vi "Timer Action Engine Auto Reset.vi"(9 "Current State":bool, 10 "Time Duration (s)":dbl, 11 "Action":T1) -> (0 "Quit Timer":bool, 1 "Clock Output":bool, 2 "Pulse Out":bool, 3 "Time Elapsed":dbl)   [LabVIEW 2021]
uses:
  Controls/Timer Actions.ctl
panel:
  # "Momentary Pulse O/P"
  # "Square Wave Pulse O/P"
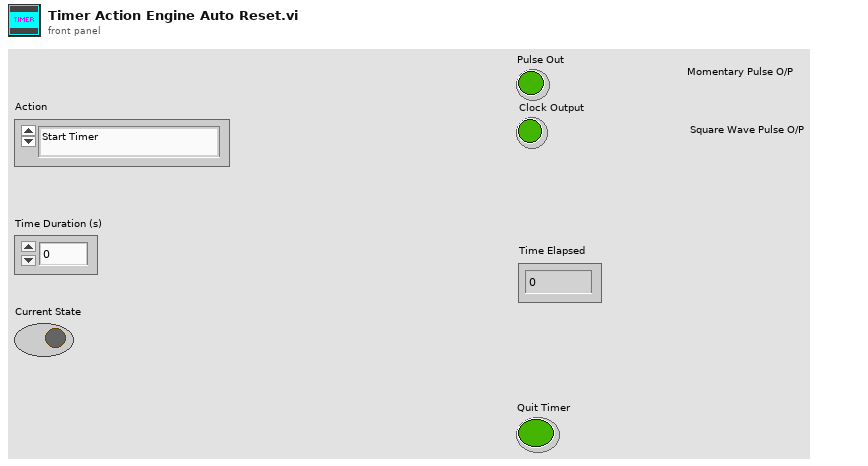
[diagram p1: front panel]
types:
  T1 = typedef "Timer Actions.ctl" = enum16{"Start Timer", "Restart Timer", "Check Timer", "Pause Timer", "Reset Timer", "Exit Timer"}
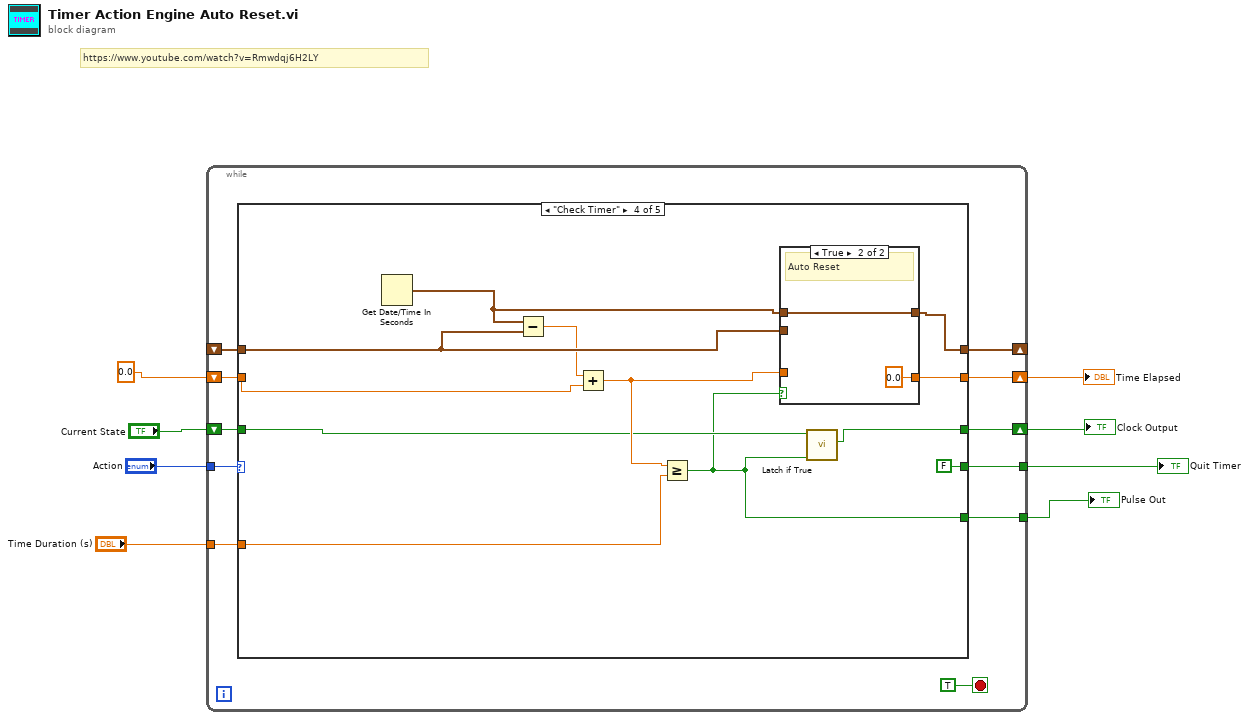
[diagram p0: block diagram]
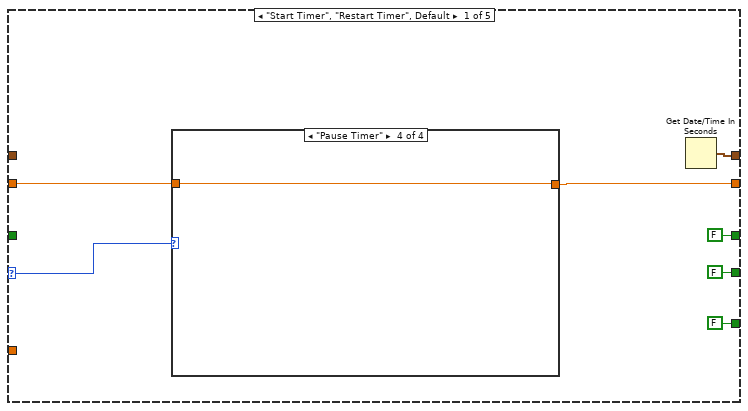
[diagram p2: hidden frame]
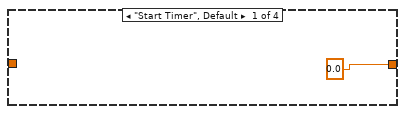
[diagram p3: hidden frame]
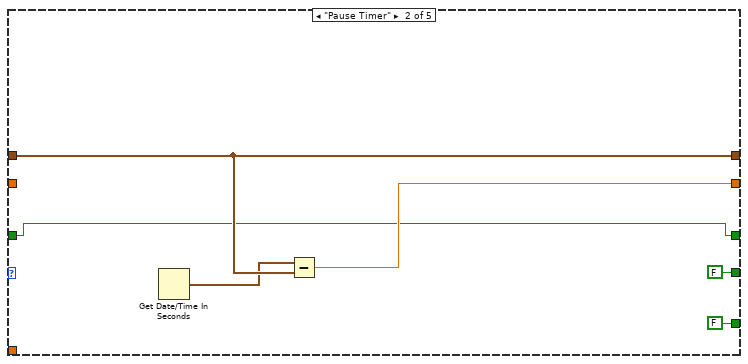
[diagram p6: hidden frame]
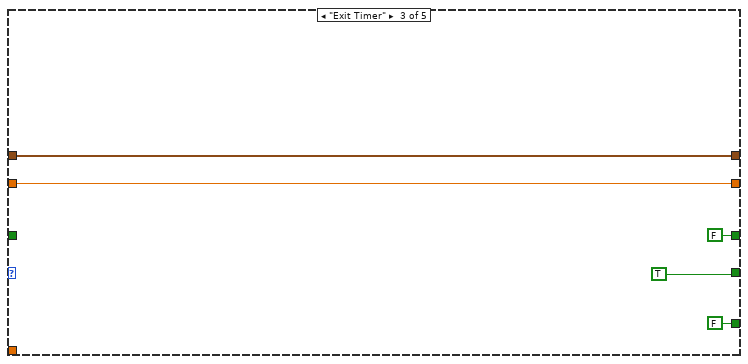
[diagram p7: hidden frame]
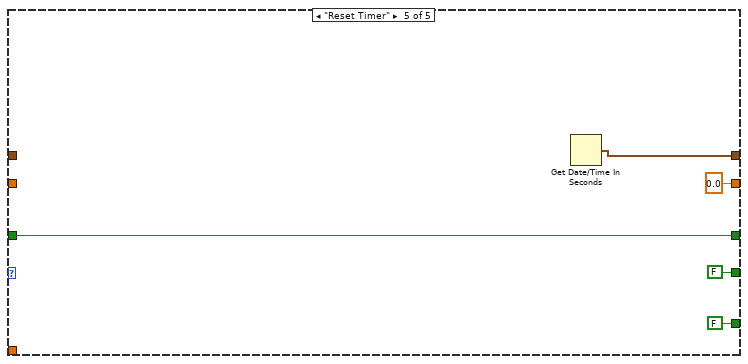
[diagram p9: hidden frame]
diagram:
  # "https://www.youtube.com/watch?v=Rmwdqj6H2LY"
  n1 = while {
    tunnel: "Action" -> [w19]
    shift-right: [w18] -> _
    shift-left: _ -> [w15]
    shift-right: [w17] -> w6
    shift-left: 0.0 ("Time Elapsed") -> [w9]
    tunnel: "Time Duration (s)" -> [w14]
    tunnel: [w13] -> w4
    shift-right: [w12] -> w3
    shift-left: "Current State" -> [w11]
    tunnel: [w10] -> w2
    stop <- TRUE stop-if-true
    n2 = case shown="\"Check Timer\"" w19 {
      selector: w19 -> [w25 _ _ _ _]
      tunnel: [w26 w36 w41 w50 w60] -> w18
      tunnel: [w24 w34 w37 w45 0.0 ("Time Elapsed")] -> w17
      tunnel: w15 -> [_ w36 w41 w51 _]
      tunnel: w14 -> [_ _ _ w53 _]
      tunnel: [FALSE FALSE TRUE FALSE FALSE] -> w13
      tunnel: [FALSE w31 FALSE w44 w59] -> w12
      tunnel: w11 -> [_ w31 _ w43 w59]
      tunnel: [FALSE FALSE FALSE w42 FALSE] -> w10
      tunnel: w9 -> [w20 _ w37 w49 _]
      frame "Start Timer", "Restart Timer", Default {
        n3 = case shown="\"Pause Timer\"" w25 {
          tunnel: [0.0 ("Time Elapsed") w28 w29 w30] -> w24
          tunnel: w20 -> [_ w28 w29 w30]
          frame "Start Timer", Default {
          }
          frame "Restart Timer" {
          }
          frame "Check Timer" {
          }
          frame "Pause Timer" {
          }
        }
        n4 = Get Date/Time In Seconds() -> (seconds since 1Jan1904=w26:timestamp)
      }
      frame "Pause Timer" {
        n5 = Get Date/Time In Seconds() -> (seconds since 1Jan1904=w35:timestamp)
        n6 = Subtract(x=w35, y=w36) -> (x-y=w34:dbl)
      }
      frame "Exit Timer" {
      }
      frame "Check Timer" {
        n7 = Get Date/Time In Seconds() -> (seconds since 1Jan1904=w47:timestamp)
        n8 = Subtract(x=w47, y=w51) -> (x-y=w48:dbl)
        n9 = Add(x=w48, y=w49) -> (x+y=w46:dbl)
        n10 = Greater Or Equal?(x=w46, y=w53) -> (x >= y?=w42:bool)
        n11 = case shown="True" w42 {
          tunnel: w51 -> [w55 _]
          tunnel: [w55 w57] -> w50
          tunnel: w47 -> [_ w57]
          tunnel: w46 -> [w54 _]
          tunnel: [w54 0.0] -> w45
          frame False {
          }
          frame True {
            # "Auto Reset"
          }
        }
        n12 = call "Latch if True.vi"("Switch State"=w42, "Current State"=w43) -> ("State Out"=w44:bool)  [unwired: 9 in]
      }
      frame "Reset Timer" {
        n13 = Get Date/Time In Seconds() -> (seconds since 1Jan1904=w60:timestamp)
      }
    }
  }
  "Quit Timer" <- w4
  "Time Elapsed" <- w6
  "Clock Output" <- w3
  "Pulse Out" <- w2
